vi "Untitled 1.vi"() -> ()   [LabVIEW 2016]
uses:
  Websockets/Opcode.ctl
  Websockets/LV WebSockets.lvlib
panel:
  out "*(type *) &x":T1
  in  "x":u8
  in  "s":bool
  out "element":bool
  out "Boolean array":bool[](array[boolean])
  out "lo(x)":u8
  out "hi(x)":u8
  out "x .and. y? 2":u8
  in  "Opcode":T1
  out "x .and. y?":u8 format="%x"
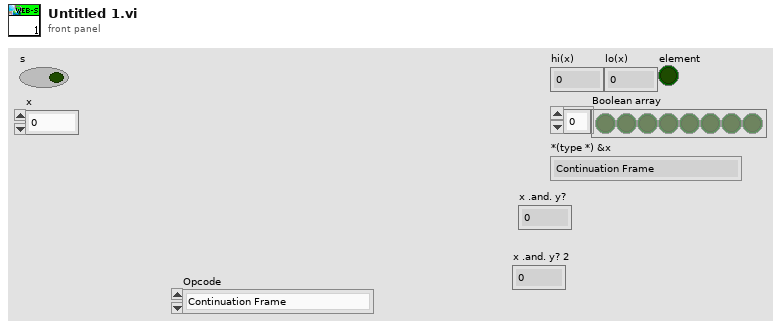
[diagram p1: front panel]
types:
  T1 = typedef "LV WebSockets.lvlib/Opcode.ctl" = enum8{"Continuation Frame", "Text Frame", "Binary Frame", "Reserved 3", "Reserved 4", "Reserved 5", "Reserved 6", "Reserved 7", "Connection Close", "Ping", "Pong", "Reserved B", "Reserved C", "Reserved D", "Reserved F"}
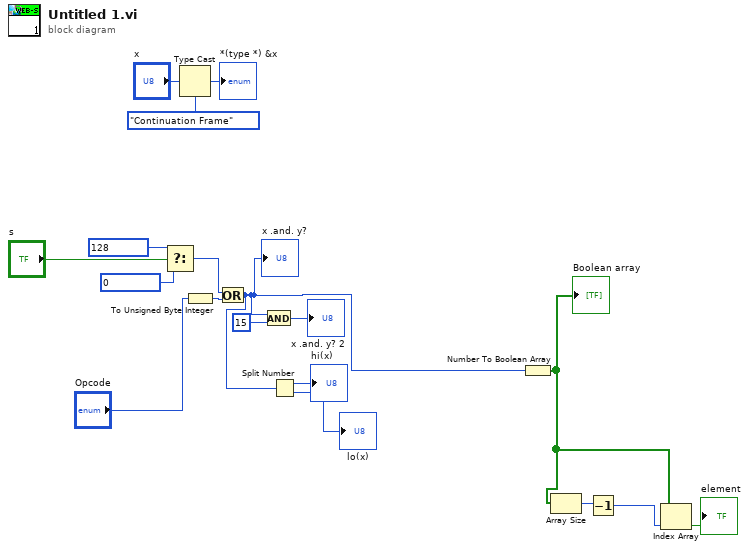
[diagram p0: block diagram]
diagram:
  n1 = Select(t=u8 128, s="s", f=u8 0) -> (s? t:f=w4:u8)
  n2 = Type Cast(type=Opcode."Continuation Frame" ("Opcode"), x="x") -> (*(type *) &x=→"*(type *) &x":T1)
  n3 = To Unsigned Byte Integer(number="Opcode") -> (unsigned 8bit integer=w17:u8)
  n4 = Or(x=w4, y=w17) -> (x .or. y?=w12:u8)
  "x .and. y?" <- w12
  n5 = And(x=w12, y=u8 15) -> (x .and. y?=→"x .and. y? 2":u8)
  n6 = Split Number(x=w12) -> (hi(x)=→"hi(x)":u8, lo(x)=→"lo(x)":u8)
  n7 = Number To Boolean Array(number=w12) -> (Boolean array=w9:bool[])
  "Boolean array" <- w9
  n8 = Array Size(array=w9) -> (size(s)=w11:i32)
  n9 = Decrement(x=w11) -> (x-1=w10:i32)
  n10 = Index Array(array=w9, index=w10) -> (element=→"element":bool)
